vi "Mouse Move.vi"(8 "error in (no error)":errorcluster, 11 "SwipeMenu in":refnum<class "SwipeMenu.lvclass">) -> (0 "error out":errorcluster, 3 "SwipeMenu out":refnum<class "SwipeMenu.lvclass">)   [LabVIEW 2019, in "SwipeMenu.lvclass"]
uses:
  SwipeMenu.lvclass
  SwipeMenu.lvclass/SwipeMenu.ctl
  <vilib>/Utility/inputDevices.llb/mouseAcquire.vi
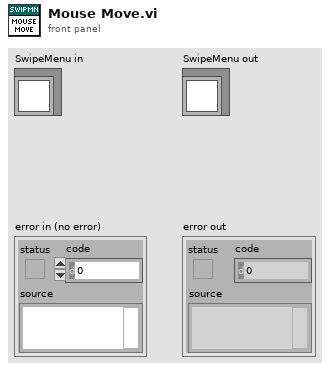
[diagram p1: front panel]
types:
  T1 = cluster{"Horizontal":i32, "Vertical":i32, "Scrolling":i32}
  T2 = typedef "SwipeMenu.lvclass/State Data.ctl" = cluster{"State":enum16{"Idle", "Mouse Nav", "Slowdown", "Button Nav"}, "Timeout":i32, "Time":timestamp, "Position":i32, "Scroll Position":i16, "Rate":dbl, "Direction":enum16{"Left", "Right"}}
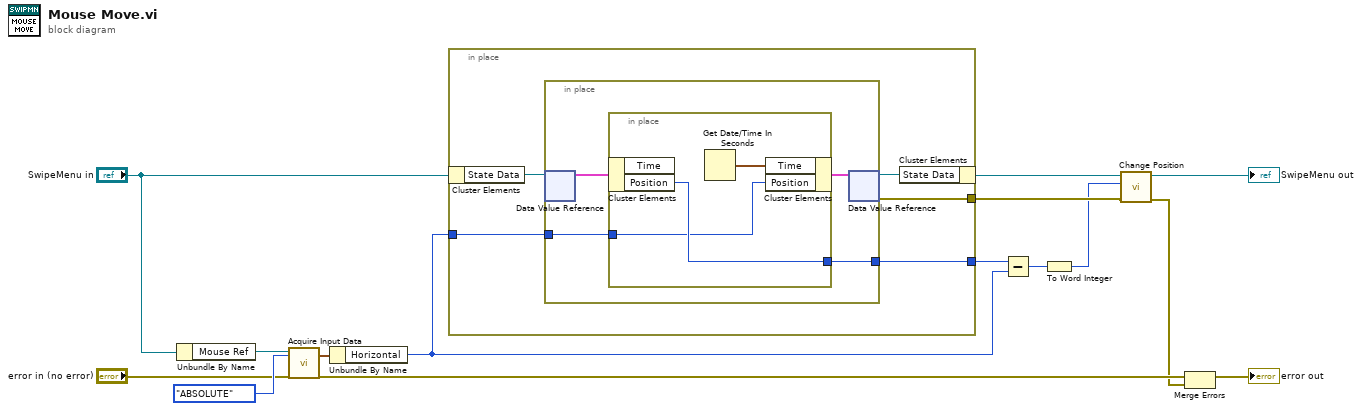
[diagram p0: block diagram]
diagram:
  n1 = Unbundle By Name("SwipeMenu in") -> ("Mouse Ref"=w13:refnum<k1>)
  n2 = call-poly <vilib>:"Acquire Input Data.vi"("device ID"=w13, "key mode"=enum16{"RELATIVE", "ABSOLUTE"}."ABSOLUTE", "error in (no error)"="error in (no error)") -> ("axis info"=w14:T1, "error out"=w12:errorcluster)  [unwired: 13 in, 2 out]
  n3 = Unbundle By Name(w14) -> ("Horizontal"=w7:i32)
  n4 = in-place {
    in-place-border: [w18] -> w11
    in-place-border: [w17] -> w3
    in-place-border: w7 -> [w16]
    n5 = in-place-cluster #1("SwipeMenu in") -> ("State Data"=w20:refnum<data-value>)
    n6 = in-place {
      in-place-border: [w24] -> w18
      in-place-border: w16 -> [w23]
      n7 = in-place-dvr #2(w20) -> (w22:T2)  [unwired: 1 out]
      n8 = in-place {
        in-place-border: [w26] -> w24
        in-place-border: w23 -> [w25]
        n9 = in-place-cluster #3(w22) -> ("Position"=w26:i32)  [unwired: 1 out]
        n10 = Get Date/Time In Seconds() -> (seconds since 1Jan1904=w27:timestamp)
        n11 = in-place-cluster #3("Time"=w27, "Position"=w25) -> (w21:T2)
      }
      n12 = in-place-dvr #2(w21) -> (w19:refnum<data-value>, w17:errorcluster)
    }
    n13 = in-place-cluster #1("State Data"=w19) -> (w5:refnum<class "SwipeMenu.lvclass">)
  }
  n14 = Subtract(x=w11, y=w7) -> (x-y=w10:i32)
  n15 = To Word Integer(number=w10) -> (16bit integer=w2:i16)
  n16 = call "Change Position.vi"("error in (no error)"=w3, "Change Position"=w2, "SwipeMenu in"=w5) -> ("error out"=w1:errorcluster, "SwipeMenu out"=→"SwipeMenu out":refnum<class "SwipeMenu.lvclass">)  [unwired: 6 in, 1 out]
  n17 = Merge Errors(w12, w1) -> (→"error out":errorcluster)
